vi "AverageTemperatures.vi"(11 "Raw Temperatures":dbl[][](array[numeric])) -> (3 "Temperatures (C)":dbl[](array[numeric]))   [LabVIEW 2012]
uses:
  <vilib>/Analysis/baseanly.llb/Mean (DBL).vi
  <vilib>/Analysis/NI_AALBase.lvlib
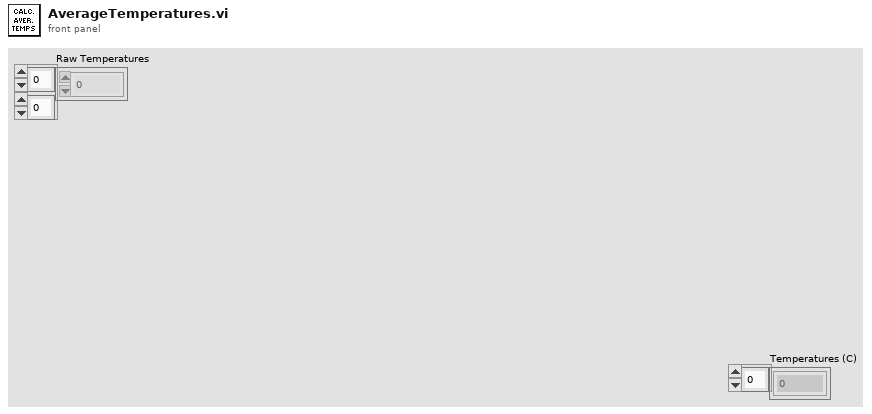
[diagram p1: front panel]
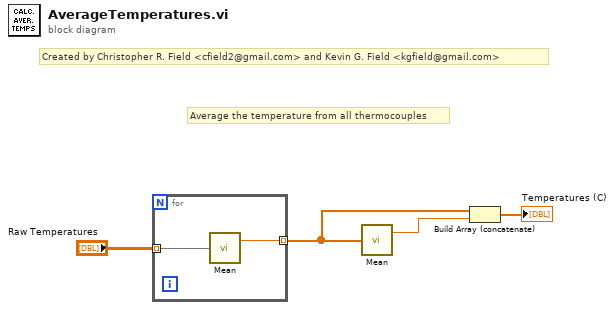
[diagram p0: block diagram]
diagram:
  # "Created by Christopher R. Field <cfield2@gmail.com> and Kevin G. Field <kgfield@gmail.com>"
  # "Average the temperature from all thermocouples"
  n1 = for {
    tunnel: "Raw Temperatures" -> [w6] mode=indexing
    tunnel: [w5] -> w3 mode=indexing
    n2 = call-poly <vilib>:"Mean.vi"("X"=w6) -> ("mean"=w5:dbl)  [unwired: 1 out]
  }
  n3 = call-poly <vilib>:"Mean.vi"("X"=w3) -> ("mean"=w2:dbl)  [unwired: 1 out]
  n4 = Build Array (concatenate)(w3, w2) -> (→"Temperatures (C)":dbl[])
